vi "Auto3 (1).vi"(0 "RobotDriveDevRef":T1, 7 "milliseconds to wait":u32=2500, 11 "error in (no error)":errorcluster) -> (2 "Hook Center 2":dbl, 3 "Initial Hook Found 2":bool, 4 "Initial Hook Center 3":dbl, 6 "Pixels to turn 2":dbl, 8 "Initial Hook Center 6":dbl, 10 "Initial Hook Found 5":bool, 12 "Hook found 2":bool, 13 "Degrees to turn 1":dbl)   [LabVIEW 2016]
uses:
  <vilib>/Rock Robotics/WPI/RobotDrive/WPI_RobotDriveDevRef.ctl
  <vilib>/Rock Robotics/WPI/MotorControl/WPI_MotorControlDeviceRef.ctl
  <vilib>/Rock Robotics/WPI/MotorControl/WPI_MotorControlType.ctl
  <vilib>/Rock Robotics/SystemInterfaces/DIO/FPGA_DIOPWMChannel.ctl
  <vilib>/Rock Robotics/WPI/PWM/WPI_PWMDeadband.ctl
  <vilib>/Rock Robotics/WPI/RobotDrive/WPI_RobotDriveArcadeDrive_Standard(NoSaturation).vi
  Robot Global Data.vi
panel:
  out "Degrees to turn 2":dbl
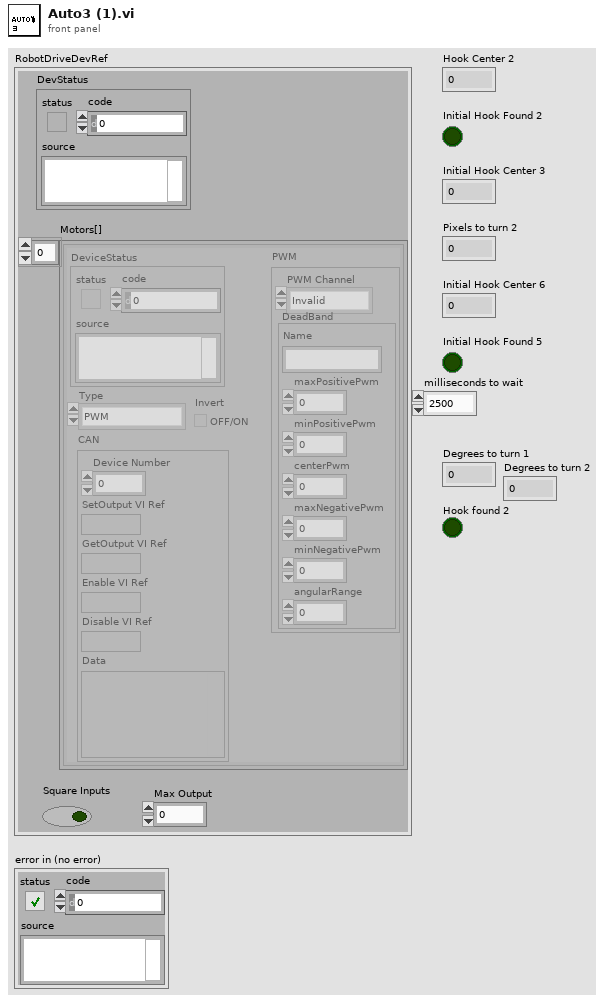
[diagram p1: front panel]
types:
  T1 = typedef "WPI_RobotDriveDevRef.ctl" = cluster{"DevStatus":errorcluster, "Motors[]":T2[], "Square Inputs":bool, "Max Output":dbl}
  T2 = typedef "WPI_MotorControlDeviceRef.ctl" = cluster{"DeviceStatus":errorcluster, "Type":T3, "PWM":cluster{"PWM Channel":T4, "DeadBand":T5}, "CAN":cluster{"Device Number":u8, "SetOutput VI Ref":variant, "GetOutput VI Ref":variant, "Enable VI Ref":variant, "Disable VI Ref":variant, "Data":variant}, "Invert":bool}
  T3 = typedef "WPI_MotorControlType.ctl" = enum16{"PWM", "CAN"}
  T4 = typedef "FPGA_DIOPWMChannel.ctl" = enum8{"PWM 0", "PWM 1", "PWM 2", "PWM 3", "PWM 4", "PWM 5", "PWM 6", "PWM 7", "PWM 8", "PWM 9", "PWM MXP 0", "PWM MXP 1", "PWM MXP 2", "PWM MXP 3", "PWM MXP 4", "PWM MXP 5", "PWM MXP 6", "PWM MXP 7", "PWM MXP 8", "PWM MXP 9", "Invalid"}
  T5 = typedef "WPI_PWMDeadband.ctl" = cluster{"Name":string, "maxPositivePwm":i32, "minPositivePwm":i32, "centerPwm":i32, "maxNegativePwm":i32, "minNegativePwm":i32, "angularRange":u16}
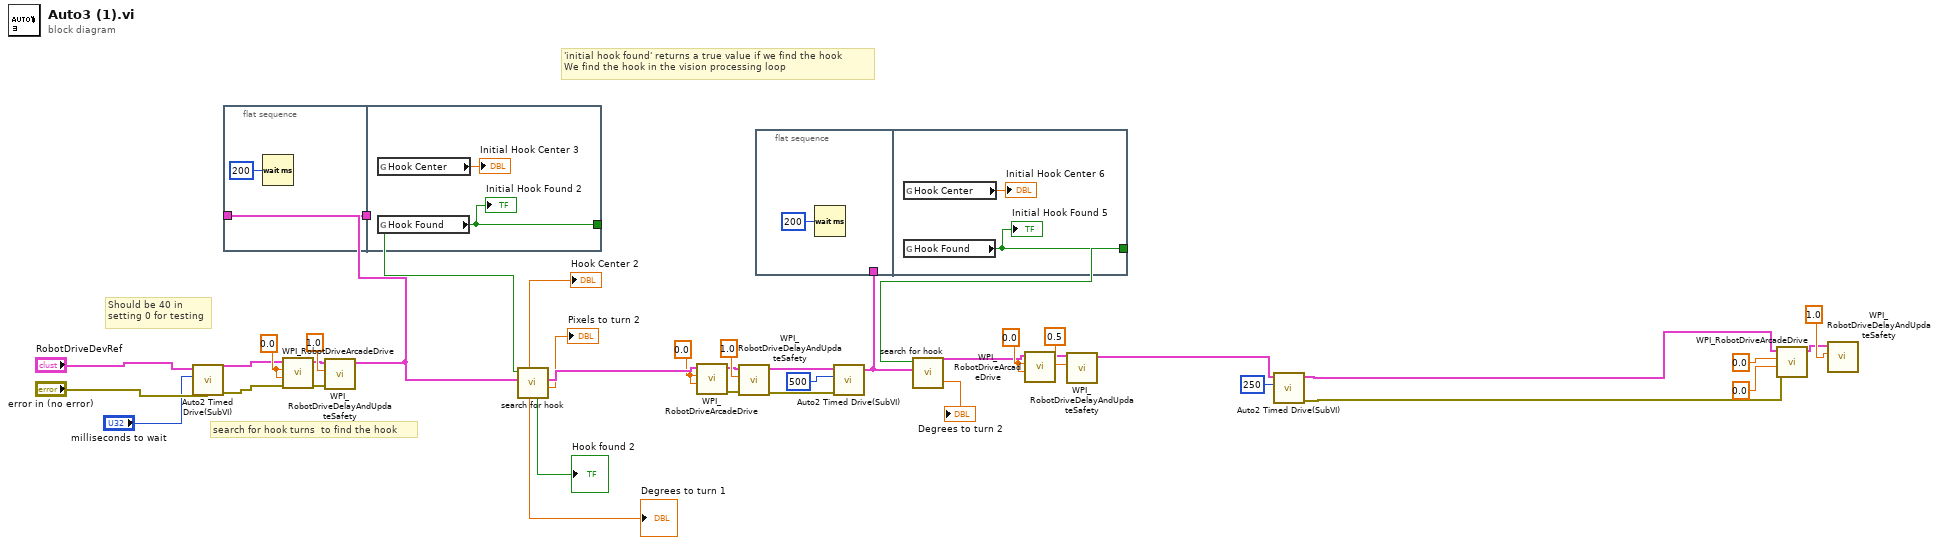
[diagram p0: block diagram]
diagram:
  w5 = 0.0 ("X axis value")
  w34 = 0.0 ("X axis value")
  w24 = 0.0 ("X axis value")
  # "'initial hook found' returns a true value if we find the hook \nWe find the hook in the vision processing loop"
  # "search for hook turns  to find the hook"
  # "Should be 40 in\nsetting 0 for testing"
  n1 = call "Auto2 Timed Drive(SubVI).vi"("error in (no error)"="error in (no error)", "milliseconds to wait"="milliseconds to wait", "RobotDriveDevRef in"="RobotDriveDevRef") -> ("error out"=w17:errorcluster, "RobotDriveDevRef out"=w18:T1)  [unwired: 7 in]
  n2 = flat-sequence {
    tunnel: w25 -> [w41]
    tunnel: [w41] -> w9
    tunnel: [w42] -> w26
    tunnel: w9 -> [_]
    frame #0 {
      n3 = Wait (ms)(milliseconds to wait=u32 200) -> ()  [unwired: 1 out]
    }
    frame #1 {
      n4 = global read "Robot Global Data.vi" "Hook Center"() -> (→"Initial Hook Center 3":dbl)
      n5 = global read "Robot Global Data.vi" "Hook Found"() -> (w42:bool)
      "Initial Hook Found 2" <- w42
    }
  }
  n6 = call-poly <vilib>:"WPI_RobotDriveArcadeDrive.vi"("error in (no error)"=w17, "Y axis value"=w24, "X axis value"=w24, "RobotDriveDevRef"=w18) -> ("error out"=w22:errorcluster, "RobotDriveDevRef"=w21:T1)  [unwired: 6 out]
  n7 = call <vilib>:"WPI_RobotDriveDelayAndUpdateSafety.vi"("error in (no error)"=w22, "Delay (s)"=1.0, "RobotDriveDevRef"=w21) -> ("RobotDriveDevRef 2"=w25:T1)  [unwired: 7 in, 1 out]
  n8 = call "search for hook.vi"("RobotDriveDevRef in"=w25, "Hook Found"=w26) -> ("Pixels to turn"=→"Pixels to turn 2":dbl, "RobotDriveDevRef out"=w35:T1, "Hook found"=→"Hook found 2":bool, "Degrees to turn"=→"Degrees to turn 1":dbl, "Hook Center"=→"Hook Center 2":dbl)  [unwired: 2 in, 3 out]
  n9 = call-poly <vilib>:"WPI_RobotDriveArcadeDrive.vi"("Y axis value"=w34, "X axis value"=w34, "RobotDriveDevRef"=w35) -> ("error out"=w32:errorcluster, "RobotDriveDevRef"=w31:T1)  [unwired: 1 in, 6 out]
  n10 = call <vilib>:"WPI_RobotDriveDelayAndUpdateSafety.vi"("error in (no error)"=w32, "Delay (s)"=1.0, "RobotDriveDevRef"=w31) -> ("error out"=w15:errorcluster, "RobotDriveDevRef 2"=w8:T1)  [unwired: 7 in]
  n11 = flat-sequence {
    tunnel: w7 -> [_]
    tunnel: [w45] -> w39
    frame #0 {
      n12 = Wait (ms)(milliseconds to wait=u32 200) -> ()  [unwired: 1 out]
    }
    frame #1 {
      n13 = global read "Robot Global Data.vi" "Hook Center"() -> (→"Initial Hook Center 6":dbl)
      n14 = global read "Robot Global Data.vi" "Hook Found"() -> (w45:bool)
      "Initial Hook Found 5" <- w45
    }
  }
  n15 = call "Auto2 Timed Drive(SubVI).vi"("error in (no error)"=w15, "milliseconds to wait"=u32 500, "RobotDriveDevRef in"=w8) -> ("RobotDriveDevRef out"=w7:T1)  [unwired: 7 in, 1 out]
  n16 = call "search for hook.vi"("RobotDriveDevRef in"=w7, "Hook Found"=w39) -> ("RobotDriveDevRef out"=w3:T1, "Degrees to turn"=→"Degrees to turn 2":dbl)  [unwired: 2 in, 6 out]
  n17 = call-poly <vilib>:"WPI_RobotDriveArcadeDrive.vi"("Y axis value"=w5, "X axis value"=w5, "RobotDriveDevRef"=w3) -> ("RobotDriveDevRef"=w2:T1)  [unwired: 1 in, 7 out]
  n18 = call <vilib>:"WPI_RobotDriveDelayAndUpdateSafety.vi"("Delay (s)"=0.5, "RobotDriveDevRef"=w2) -> ("RobotDriveDevRef 2"=w1:T1)  [unwired: 8 in, 1 out]
  n19 = call "Auto2 Timed Drive(SubVI).vi"("milliseconds to wait"=u32 250, "RobotDriveDevRef in"=w1) -> ("error out"=w11:errorcluster, "RobotDriveDevRef out"=w12:T1)  [unwired: 8 in]
  n20 = call-poly <vilib>:"WPI_RobotDriveArcadeDrive.vi"("error in (no error)"=w11, "Y axis value"=0.0 ("X axis value"), "X axis value"=0.0, "RobotDriveDevRef"=w12) -> ("RobotDriveDevRef"=w37:T1)  [unwired: 7 out]
  n21 = call <vilib>:"WPI_RobotDriveDelayAndUpdateSafety.vi"("Delay (s)"=1.0, "RobotDriveDevRef"=w37) -> ()  [unwired: 8 in, 2 out]
